vi "EEG_2021_099 1D arrays.vi"() -> ()   [LabVIEW 2022 SP3]
panel:
  out "Array 4":bool[](array[boolean])
  in  "Array 3":bool[](array[boolean])
  out "Array 2":dbl[](array[slide]) scale=0.0..10.0
  in  "Array":dbl[](array[numeric])
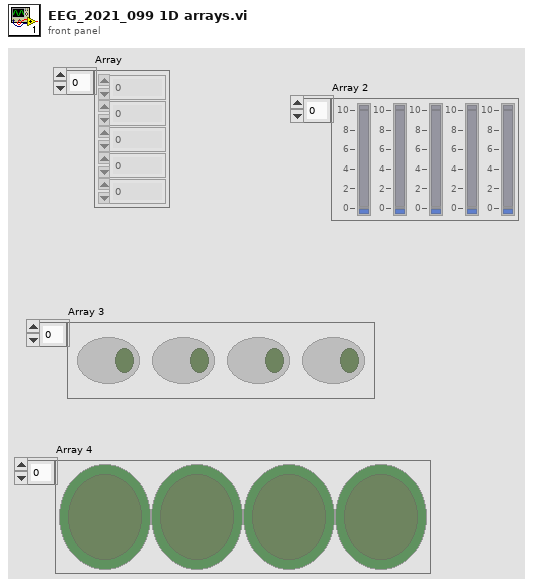
[diagram p1: front panel]
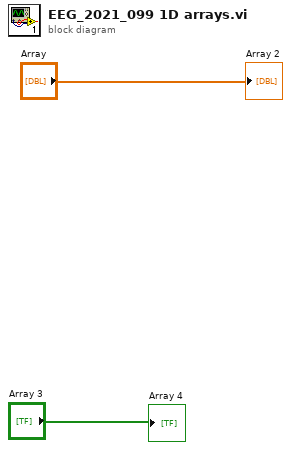
[diagram p0: block diagram]
diagram:
  "Array 2" <- "Array"
  "Array 4" <- "Array 3"
